vi "ABC.vi"(0 "Image In":T3, 1 "ROI Descriptor (OCR/OCV 1)":T2={"Global Rectangle"=[100, 100, 250, 150], "Contours"=[{"ID"=enum."External", "Type"=3, "Coordinates"=[100, 100, 250, 150]}]} {"Contours"."Type" items=["No Selection", "Point", "Line", "Rectangle", "Oval", "Polygon", "Freehand Region", "Annulus", "Unused2", "Unused3", "Broken Line", "Freehand Line", "Rotated Rectangle"]}, 2 "File Path (OCR/OCV 1)":path=path "C:/Users/miagu/OneDrive/Escritorio/NUMBER.abc", 3 "Parameters (OCR/OCV 1)":T1={"Threshold Data"={"Method"=enum."Uniform", "Looking for"=1, "Color Mode"=0, "Kernel Size"={"Width"=32, "Height"=32}, "Ranges"=[{"Min"=1, "Max"=255}]}, "Reject Border"=TRUE, "Number Of Erosions"=0, "Size & Spacing"={"Segment Algorithm"=0, "Min Bounding Rect Width"=1, "Max Bounding Rect Width"=65536, "Min Bounding Rect Height"=1, "Max Bounding Rect Height"=65536, "Min Character Size"=20, "Max Character Size"=65536, "Min Char Spacing"=1, "Max Horiz Element Spacing"=1, "Max Vert Element Spacing"=0, "Max Space Distance"=65536}, "Read Options"={"Read Strategy"=1, "Read Resolution"=2, "Scale Dependant"=FALSE, "Aspect Ratio"=400, "Acceptance Level"=700, "Substitution Character"="?", "MultiLine"=TRUE}, "Valid Characters"=[], "Use Text Pattern"=FALSE, "Orientation"=0, "# Lines Expected"=0, "Number of Blocks"=4} {"Threshold Data"."Looking for" items=["Light on Dark", "Dark on Light"]; "Threshold Data"."Color Mode" items=["RGB", "HSL", "HSV", "HSI"]; "Size & Spacing"."Segment Algorithm" items=["None", "Shortest Segment", "Legacy Auto Split"]; "Read Options"."Read Strategy" items=["Aggressive", "Conservative"]; "Read Options"."Read Resolution" items=["Low", "Medium", "High"]; "Valid Characters"."Pre-defined characters" items=["Any Character", "User-defined Characters", "Alphabetic", "Alphanumeric", "Uppercase Letters", "Lowercase Letters", "Decimal Digits", "Hexadecimal Digits", "Pattern", "Force Space"]; "Orientation" items=["Baseline inside", "Baseline outside"]}, 7 "error in":errorcluster) -> (20 "Image Out":T3, 21 "String (OCR/OCV 1)":string, 27 "error out":errorcluster)   [LabVIEW 2023]
uses:
  <vilib>/vision/Image Controls.llb/IMAQ Image.ctl
  <vilib>/vision/NI_Vision_Development_Module.lvlib
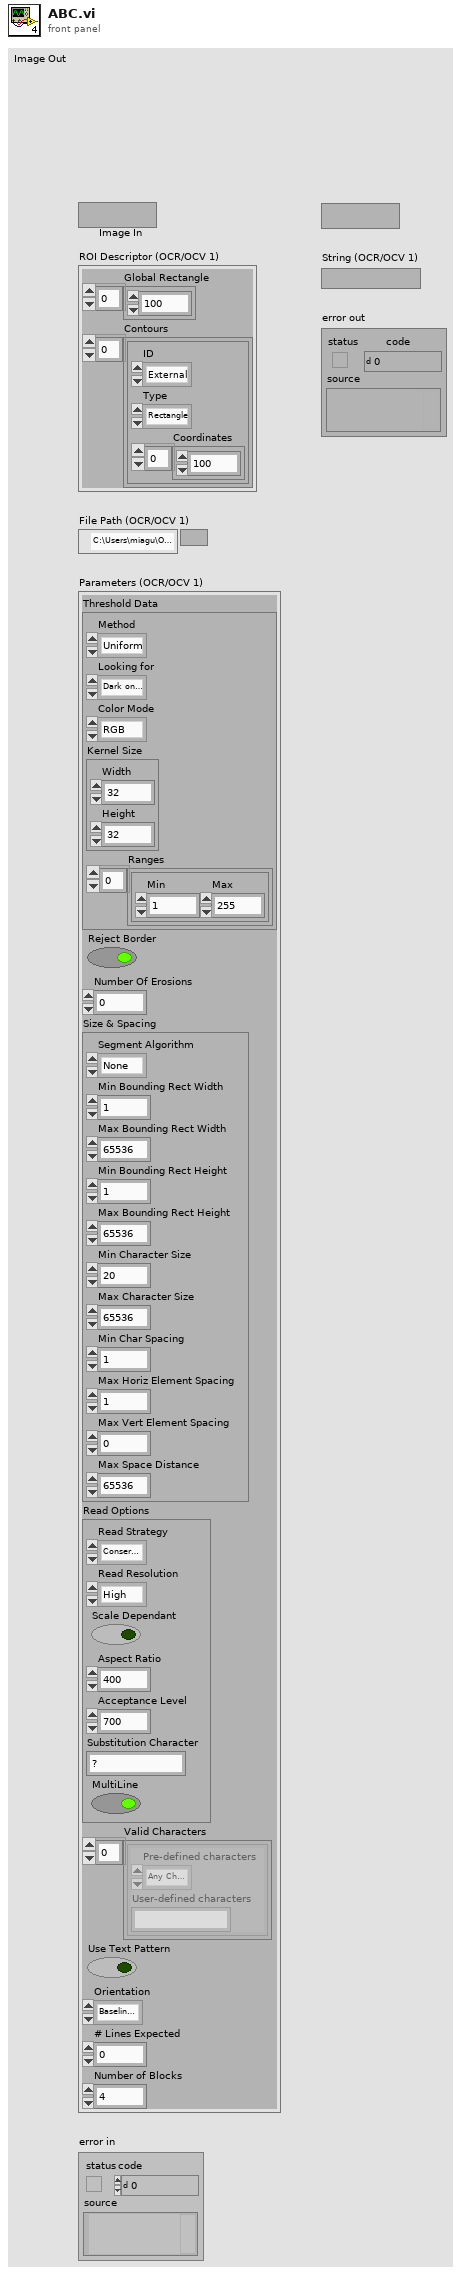
[diagram p1: front panel]
types:
  T1 = cluster{"Threshold Data":cluster{"Method":enum16{"Fixed Range", "Uniform", "Linear", "Non Linear", "Local", "Color"}, "Looking for":u32, "Color Mode":u32, "Kernel Size":cluster{"Width":i32, "Height":i32}, "Ranges":cluster{"Min":i32, "Max":i32}[]}, "Reject Border":bool, "Number Of Erosions":i32, "Size & Spacing":cluster{"Segment Algorithm":u16, "Min Bounding Rect Width":i32, "Max Bounding Rect Width":i32, "Min Bounding Rect Height":i32, "Max Bounding Rect Height":i32, "Min Character Size":i32, "Max Character Size":i32, "Min Char Spacing":i32, "Max Horiz Element Spacing":i32, "Max Vert Element Spacing":i32, "Max Space Distance":i32}, "Read Options":cluster{"Read Strategy":i32, "Read Resolution":i32, "Scale Dependant":bool, "Aspect Ratio":i32, "Acceptance Level":i32, "Substitution Character":string, "MultiLine":bool}, "Valid Characters":cluster{"Pre-defined characters":i32, "User-defined characters":string}[], "Use Text Pattern":bool, "Orientation":u32, "# Lines Expected":u32, "Number of Blocks":i32}
  T2 = cluster{"Global Rectangle":i32[], "Contours":cluster{"ID":enum32{"External", "Internal"}, "Type":u32, "Coordinates":i32[]}[]}
  T3 = typedef "IMAQ Image.ctl" = refnum<image>
  T4 = typedef "IMAQ OCR Session.ctl" = refnum<k1>
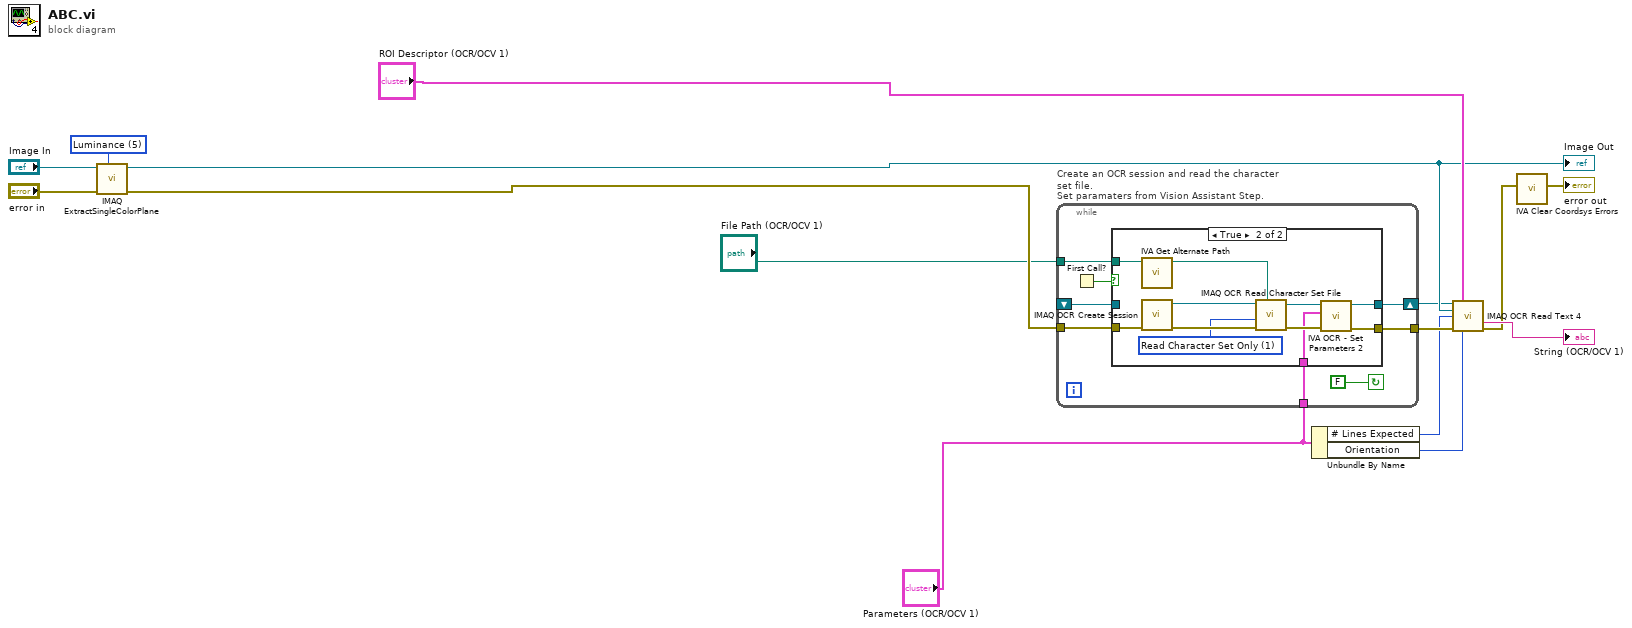
[diagram p0: block diagram]
diagram:
  w15 = 5 items=["Red", "Green", "Blue", "Hue", "Saturation", "Luminance", "Value", "Intensity"] ("Color Plane")
  n1 = call "IMAQ ExtractSingleColorPlane"("Color Plane"=w15, "error in (no error)"="error in", "Image Src"="Image In") -> ("error out"=w12:errorcluster, "Image Dst Out"=w8:T3)  [unwired: 1 in, 6 out]
  "Image Out" <- w8
  n2 = while "Create an OCR session and read the character set file.\nSet paramaters from Vision Assistant Step." {
    shift-right: [w20] -> w5
    shift-left: _ -> [w19]
    tunnel: w12 -> [w22]
    tunnel: "Parameters (OCR/OCV 1)" -> [w18]
    tunnel: "File Path (OCR/OCV 1)" -> [w17]
    tunnel: [w16] -> w6
    stop <- FALSE continue-if-true
    n3 = First Call?() -> (First Call?: T/F=w21:bool)
    n4 = case shown="True" w21 {
      tunnel: w17 -> [_ w29]
      tunnel: w22 -> [w24 w33]
      tunnel: [w25 w31] -> w20
      tunnel: [w24 w30] -> w16
      tunnel: w18 -> [_ w26]
      tunnel: w19 -> [w25 _]
      frame False {
      }
      frame True {
        w34 = 1 items=["Read All", "Read Character Set Only", "Read Properties Only"] ("Read Options")
        n5 = call <vilib>:"IVA Get Alternate Path.vi"("Path In"=w29) -> ("Path Out"=w28:path)  [unwired: 10 out]
        n6 = call "IMAQ OCR Create Session"("error in (no error)"=w33) -> ("error out"=w35:errorcluster, "IMAQ OCR Session"=w36:T4)  [unwired: 9 out]
        n7 = call "IMAQ OCR Read Character Set File"("File Path"=w28, "error in (no error)"=w35, "Read Options"=w34, "IMAQ OCR Session"=w36) -> ("error out"=w32:errorcluster, "IMAQ OCR Session (dup)"=w27:T4)  [unwired: 1 in, 5 out]
        n8 = call <vilib>:"IVA OCR - Set Parameters 2.vi"("error in (no error)"=w32, "Parameters"=w26, "IMAQ OCR Session"=w27) -> ("error out"=w30:errorcluster, "IMAQ OCR Session Out"=w31:T4)  [unwired: 7 in]
      }
    }
  }
  n9 = Unbundle By Name("Parameters (OCR/OCV 1)") -> ("# Lines Expected"=w3:u32, "Orientation"=w4:u32)
  n10 = call "IMAQ OCR Read Text 4"("IMAQ OCR Session"=w5, "ROI Descriptor"="ROI Descriptor (OCR/OCV 1)", "Image"=w8, "Number of Lines Requested"=w3, "error in (no error)"=w6, "Orientation"=w4) -> ("Read String"=→"String (OCR/OCV 1)":string, "error out"=w2:errorcluster)  [unwired: 8 out]
  n11 = call <vilib>:"IVA Clear Coordsys Errors.vi"("error in (no error)"=w2) -> ("error out"=→"error out":errorcluster)  [unwired: 10 in]
